vi "Problem 15 - backtracking-optimised.vi"(8 "error in (no error)":errorcluster) -> (0 "error out":errorcluster)   [LabVIEW 2021, in "Project Euler.lvlib"]
uses:
  Project Euler.lvlib
  lattice_path_node.ctl
  lattice_path_direction.ctl
  Utilities/Named Timers/Named Timers.lvlib
panel:
  out "no_of_routes":i32
  out "destination":T1={"position"={"i"=2, "j"=2}, "unexplored children"=[]}
  in  "start":T1={"position"={"i"=0, "j"=0}, "unexplored children"=[enum."to the right", enum."downwards"]}
  out "Loop iteration":i32
  in  "Dev: stop early":bool
  out "no. of columns":i32
  out "no. of rows":i32
  out "map\n2D array of nodes\n(n) x (n) size":T1[][](array[typedef])
  in  "n (number of nodes on a side)":i32=3
  out "Answer":string
  out "Total execution time (ms)":u32
  # "Output\nOutputs of the VI"
  # "Description\n\nBlank VI with error handling case. \n\nSummarize the use of this VI in this space."
  # "Development\ncontrols/indicators useful for development and testing, but which are not outputs of the VI"
  # "Input\nInputs to the VI"
  # "Execution time benchmarking\nFirst implementation:\n\n20x20 grid (21 nodex x 21 nodes):\n125,059 routes found in 506,856 ms -> 4.05 ms to find one route (one average)"
  # "We take n = 8 nodes (grid = 7) as our benchmark.\n\n3,432 routes when n = 8\n\nTime taken (ms)\n\n1. 1100\n2. 1124 \n3. 1116 \n\nimplemented some optimizations\n1. 1038\n2. 1067\n3. 1017\n4. 1017\n5. 1017\n\nimplemented some optimizations:\n- stop if backtracked to start node. This is expected to half execution time.\n1. 521\n2. 527\n3. 517\n4. 533\n5. 519\n\nimplemented some optimizations:\n- restarted LabVIEW after it hanged\n- replaced \"Delete Array Element\" with \"Index Array Subset\"\n1. 71\n2. 78\n3. 82\n4. 77\n5. 66\n\n- replaced \"Index Array Subset\" with \"Delete Array Element\" (back). DAE is faster than ASB in this case.\n1. 51 \n2. 44\n3. 52\n4. 53\n5. 55\n- implemented \"In Place Element Structure\" inside \"find next node.vi\". This subVI executes every iteration of the while loop, so may have a significant effect (10% decrease in exec time). Actual measurements:\n1. 448\n2. 457\n3. 468\n4. 460\n5. 450\n- restarted LabVIEW. Restarting LabVIEW has the single biggest effect on exec time. Why?\n1. 57\n2. 48\n3. 48\n4. 60\n5. 49"
  # "n = 9; 168 ms\nn= 10; 616 ms\nn =11; 2,336; non-optimised time = 8,807. Four-fold optimisation (two-fold in one go, the other factor of two compounded from several optimisations)\n\nn =12; 9119; 705,432 routes\nn =13;\n\nn=14; finished;\n10,400,600 found in 145,041 ms\nAverage: 71.71 routes per ms\n\n----\n\nn=21; stopped early.\n40,014,690 routes found (40 million)\nin\n1,458,759 ms (24.3 minutes)\nAverage: 27.43 routes found per millisecond"
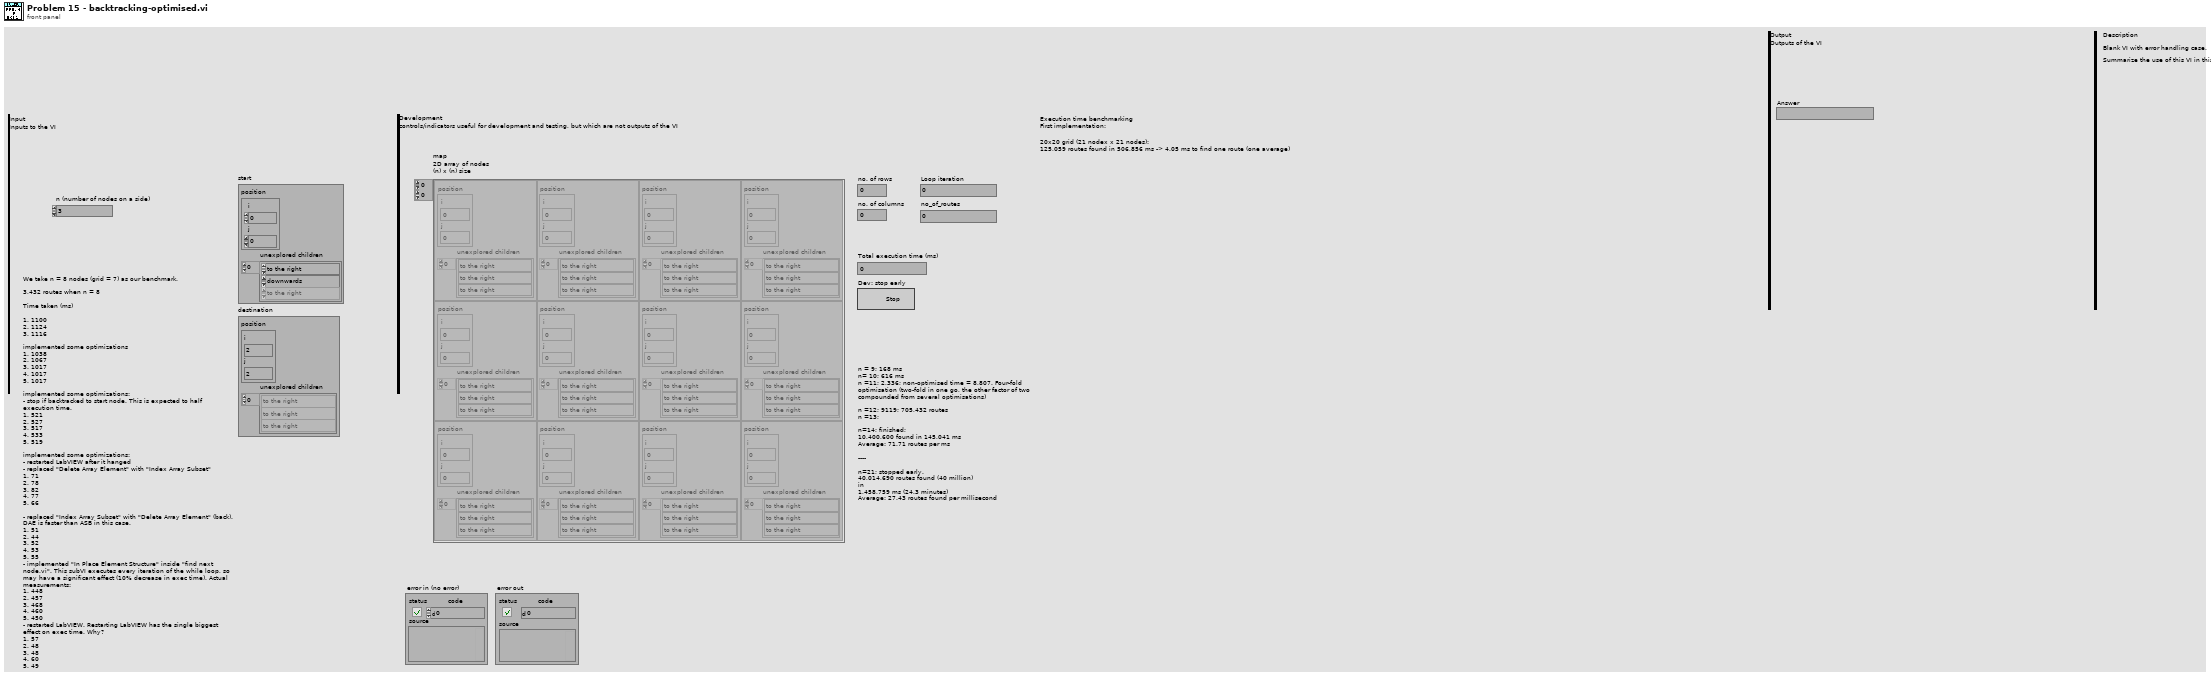
[diagram p1: front panel]
types:
  T1 = typedef "Project Euler.lvlib/lattice_path_node.ctl" = cluster{"position":cluster{"i":i32, "j":i32}, "unexplored children":T2[]}
  T2 = typedef "Project Euler.lvlib/lattice_path_direction.ctl" = enum16{"to the right", "downwards"}
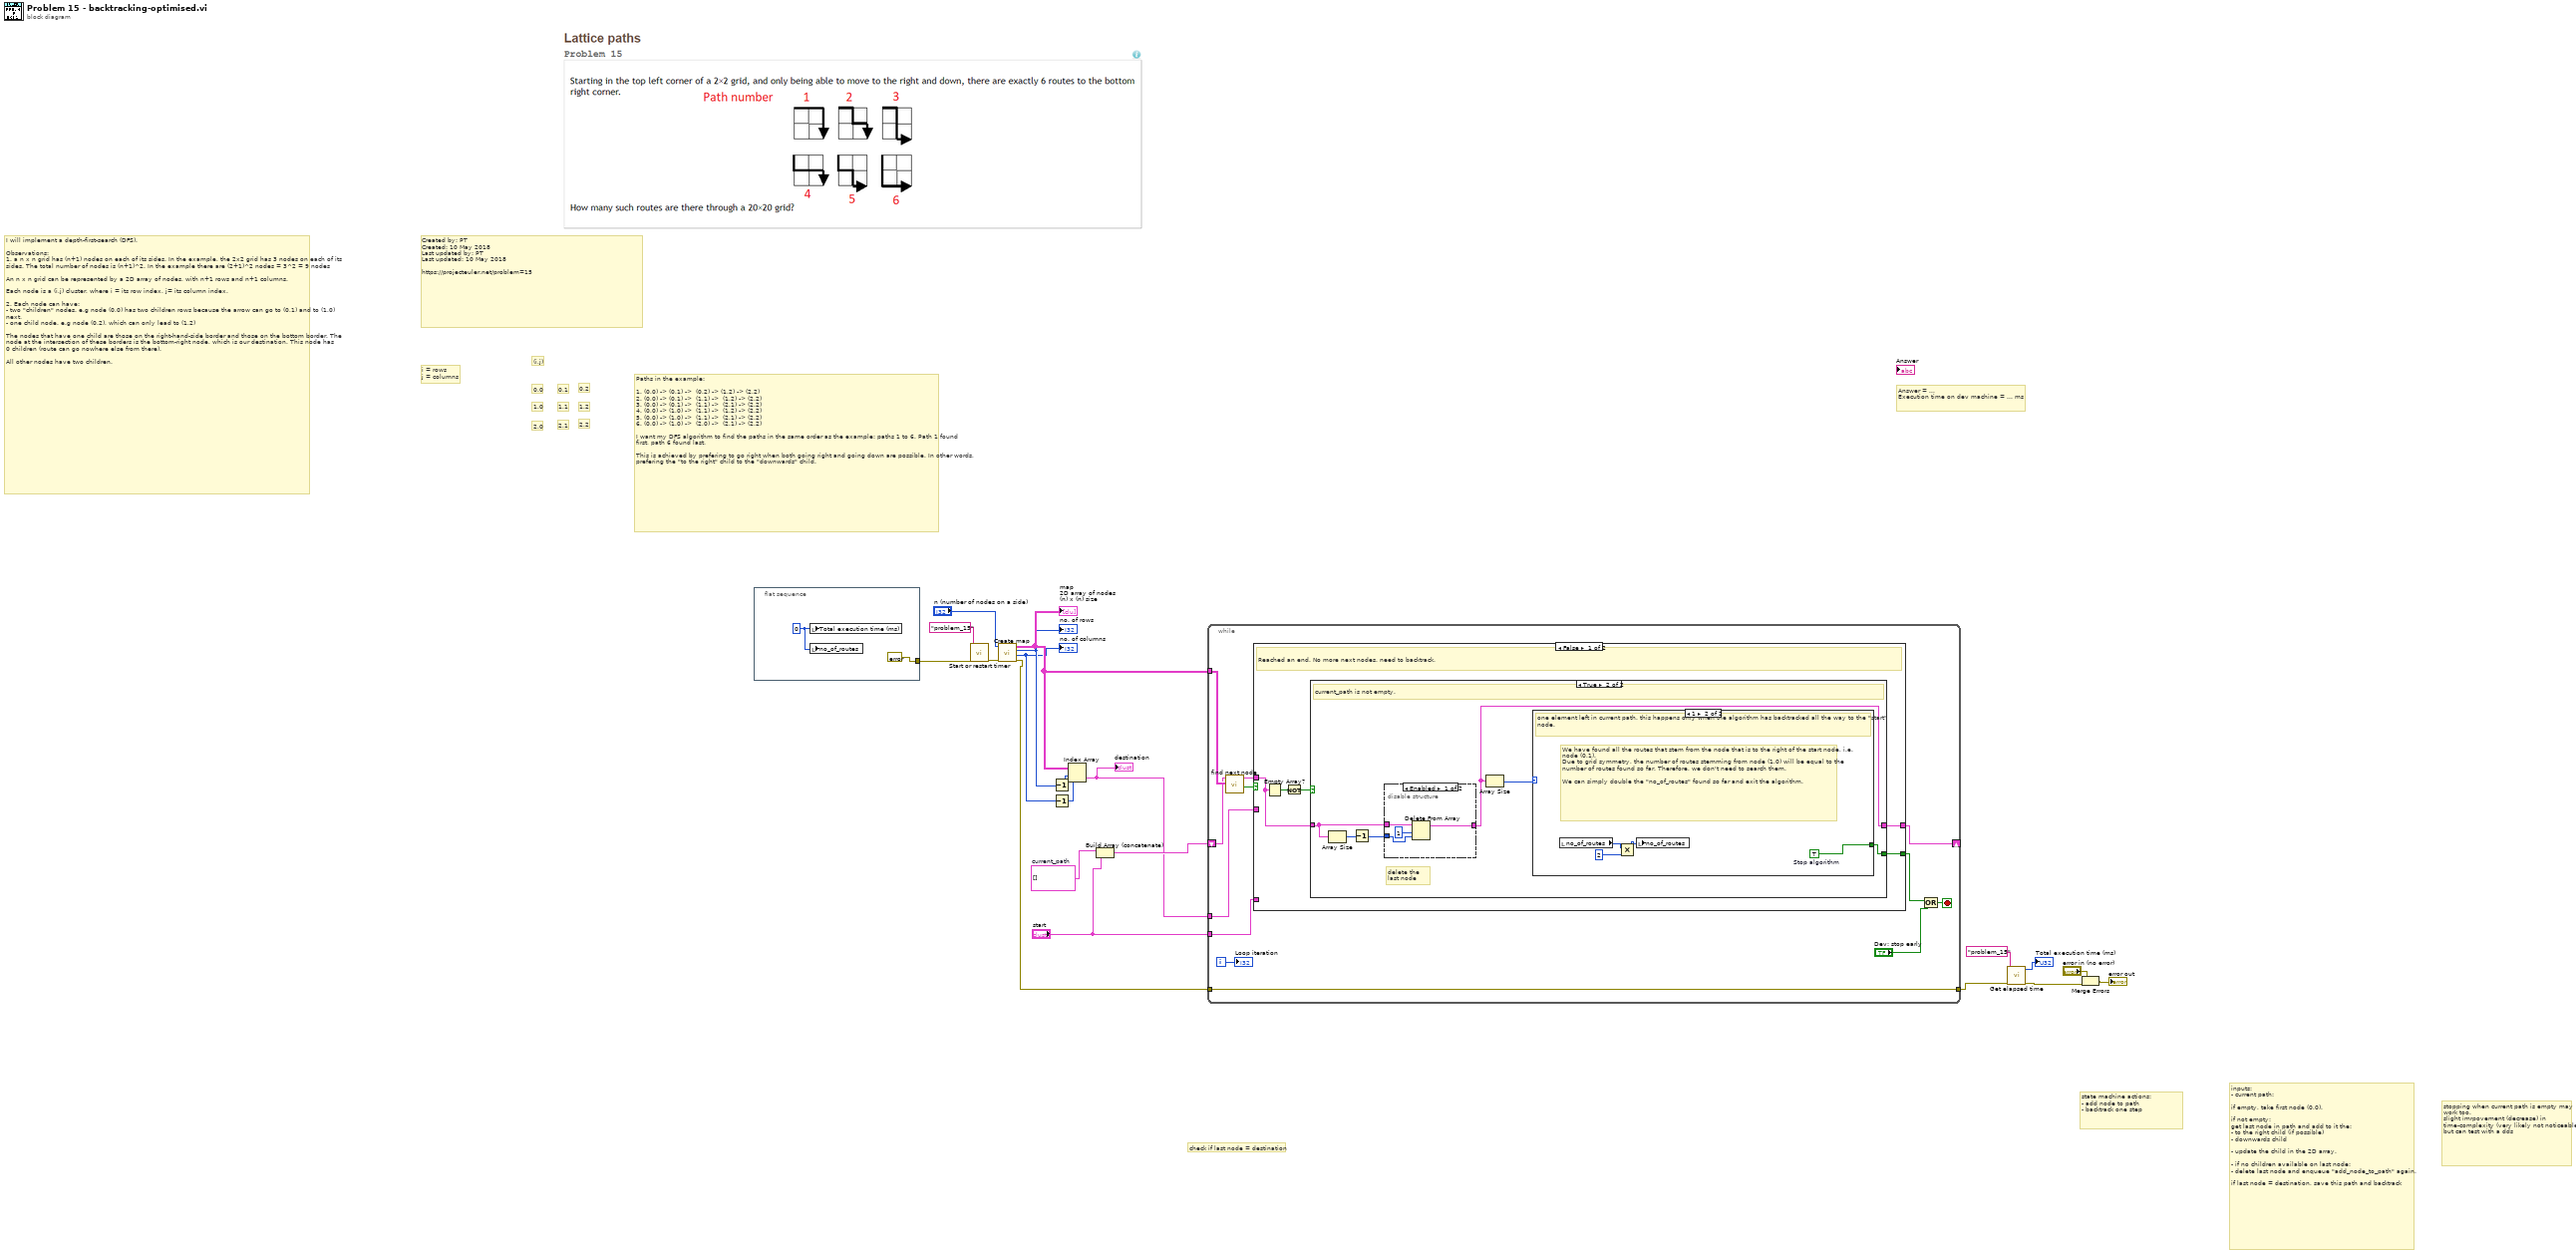
[diagram p0: block diagram]
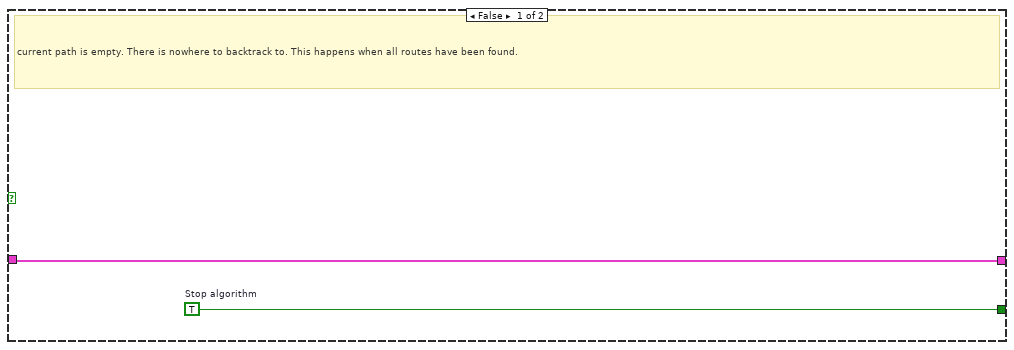
[diagram p2: hidden frame]
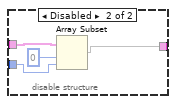
[diagram p3: hidden frame]
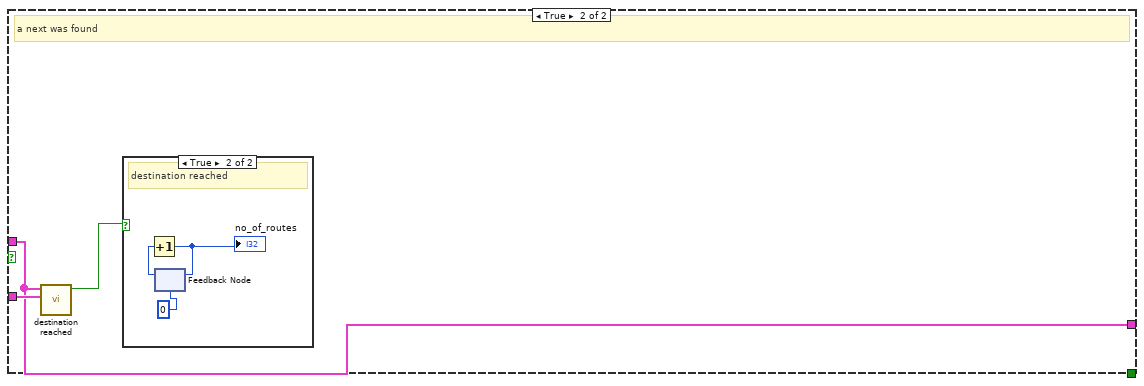
[diagram p5: hidden frame]
diagram:
  w16 = T1[] []  # current_path
  # "stopping when current path is empty may work too.\nslight imrpovement (decrease) in time-complexity (very likely not noticeable), but can test with a dds"
  # "check if last node = destination"
  # "inputs:\n- current path:\n\nif empty, take first node (0,0).\n\nif not empty:\nget last node in path and add to it the:\n- to the right child (if possible)\n- downwards child\n\n- update the child in the 2D array.\n\n- if no children available on last node:\n- delete last node and enqueue \"add_node_to_path\" again.\n\nif last node = destination, save this path and backtrack"
  # "state machine actions:\n- add node to path\n- backtrack one step"
  # "Paths in the example:\n\n1. (0,0) -> (0,1) ->  (0,2) -> (1,2) -> (2,2)\n2. (0,0) -> (0,1) ->  (1,1) ->  (1,2) -> (2,2)\n3. (0,0) -> (0,1) ->  (1,1) ->  (2,1) -> (2,2)\n4. (0,0) -> (1,0) ->  (1,1) ->  (1,2) -> (2,2)\n5. (0,0) -> (1,0) ->  (1,1) ->  (2,1) -> (2,2)\n6. (0,0) -> (1,0) ->  (2,0) ->  (2,1) -> (2,2)\n\nI want my DFS algorithm to find the paths in the same order as the example: paths 1 to 6. Path 1 found first, path 6 found last.\n\nThis is achieved by prefering to go right when both going right and going down are possible. In other words, prefering the \"to the right\" child to the \"downwards\" child."
  # "2,2"
  # "2,1"
  # "1,2"
  # "1,1"
  # "0,2"
  # "0,1"
  # "2,0"
  # "(i,j)"
  # "i = rows\nj = columns"
  # "1,0"
  # "0,0"
  # "I will implement a depth-first-search (DFS).\n\nObservations:\n1. a n x n grid has (n+1) nodes on each of its sides. In the example, the 2x2 grid has 3 nodes on each of its sides. The total number of nodes is (n+1)^2. In the example there are (2+1)^2 nodes = 3^2 = 9 nodes\n\nAn n x n grid can be represented by a 2D array of nodes, with n+1 rows and n+1 columns.\n\nEach node is a (i,j) cluster, where i = its row index, j= its column index.\n\n2. Each node can have:\n- two \"children\" nodes. e.g node (0,0) has two children rows because the arrow can go to (0,1) and to (1,0) next.\n- one child node. e.g node (0,2), which can only lead to (1,2)\n\nThe nodes that have one child are those on the right-hand-side border and those on the bottom border. The node at the intersection of these borders is the bottom-right node, which is our destination. This node has 0 children (route can go nowhere else from there).\n\nAll other nodes have two children."
  # "Answer = ... \nExecution time on dev machine = ... ms"
  # "Created by: PT\nCreated: 10 May 2018\nLast updated by: PT\nLast updated: 10 May 2018\n\nhttps://projecteuler.net/problem=15"
  n1 = flat-sequence {
    tunnel: [w22] -> _
    tunnel: [w22] -> w17
    frame #0 {
      w22 = errorcluster {"status"=FALSE, "code"=0, "source"=""} ("error constant")
      w21 = u32 0 ("Total execution time (ms)")
      n2 = local write "Total execution time (ms)"(w21) -> ()
      n3 = local write "no_of_routes"(w21) -> ()
    }
  }
  n4 = call "Start or restart timer.vi"("error in (no error)"=w17, "Timer name"="problem_15") -> ("error out"=w6:errorcluster)  [unwired: 9 in]
  n5 = call "Create map.vi"("error in (no error)"=w6, "n (number of nodes on a side)"="n (number of nodes on a side)") -> ("error out"=w3:errorcluster, "no. of columns"=w4:i32, "no. of rows"=w5:i32, "map\n2D array of nodes\n(n) x (n) size"=w8:T1[][])  [unwired: 6 in]
  "map\n2D array of nodes\n(n) x (n) size" <- w8
  "no. of rows" <- w5
  "no. of columns" <- w4
  n6 = Decrement(x=w5) -> (x-1=w11:i32)
  n7 = Decrement(x=w4) -> (x-1=w10:i32)
  n8 = Index Array(array=w8, index (row)=w11, index (col)=w10) -> (element=w9:T1)
  "destination" <- w9
  n9 = Build Array (concatenate)(w16, "start") -> (w12:T1[])
  n10 = while {
    shift-right: [w28] -> _
    shift-left: w12 -> [w30]
    tunnel: w8 -> [w31]
    tunnel: w9 -> [w29]
    tunnel: w3 -> [w24]
    tunnel: [w24] -> w2
    tunnel: "start" -> [w23]
    i -> [w32]
    stop <- w33 stop-if-true
    n11 = call "find next node.vi"("map"=w31, "current_path in"=w30) -> ("T = a next node was found"=w26:bool, "current_path out"=w25:T1[])  [unwired: 6 in, 2 out]
    n12 = case shown="False" w26 {
      tunnel: w25 -> [w37 w60]
      tunnel: w29 -> [_ w61]
      tunnel: [w36 _] -> w27
      tunnel: [w35 w60] -> w28
      tunnel: w23 -> [_ _]
      frame False {
        # "Reached an end. No more next nodes. need to backtrack."
        n13 = Empty Array?(array=w37) -> (empty?=w39:bool)
        n14 = Not(x=w39) -> (.not. x?=w38:bool)
        n15 = case shown="True" w38 {
          tunnel: w37 -> [w41 w43]
          tunnel: [w41 w45] -> w35
          tunnel: [w40 w44] -> w36
          frame False {
            w40 = TRUE  # Stop algorithm
            # "current path is empty. There is nowhere to backtrack to. This happens when all routes have been found."
          }
          frame True {
            # "delete the last node"
            # "current_path is not empty."
            n16 = Array Size(array=w43) -> (size(s)=w47:i32)
            n17 = Decrement(x=w47) -> (x-1=w42:i32)
            n18 = disable-structure shown="Enabled" {
              disable-tunnel: [w50 w53] -> w45
              disable-tunnel: w43 -> [w49 w54]
              disable-tunnel: w42 -> [w48 w52]
              frame Enabled {
                n19 = Delete From Array "Delete From Array"(array=w49, length=1, index=w48) -> (array with subset deleted=w50:T1[])  [unwired: 1 out]
              }
              frame Disabled {
                n20 = Array Subset(array=w54, index=0, length=w52) -> (w53:T1[])
              }
            }
            n21 = Array Size(array=w45) -> (size(s)=w46:i32)
            n22 = case shown="1" w46 {
              tunnel: [_ w59] -> w44
              frame Default {
                # "we have not backtracked to the \"start\" node yet"
              }
              frame 1 {
                w59 = TRUE  # Stop algorithm
                # "We have found all the routes that stem from the node that is to the right of the start node, i.e. node (0,1).\nDue to grid symmetry, the number of routes stemming from node (1,0) will be equal to the number of routes found so far. Therefore, we don't need to search them.\n\nWe can simply double the \"no_of_routes\" found so far and exit the algorithm."
                # "one element left in current path. this happens only when the algorithm has backtracked all the way to the \"start\" node."
                n23 = local read "no_of_routes"() -> (w58:i32)
                n24 = Multiply(x=w58, y=2) -> (x*y=w56:i32)
                n25 = local write "no_of_routes"(w56) -> ()
              }
            }
          }
        }
      }
      frame True {
        # "a next was found"
        n26 = call "destination reached.vi"("destination"=w61, "current_path"=w60) -> ("T = destination has been reached"=w62:bool)  [unwired: 8 in, 1 out]
        n27 = case shown="True" w62 {
          frame False {
            # "destination not reached yet"
          }
          frame True {
            # "destination reached"
            n28 = feedback #1(0) -> (w65:i32)
            n29 = Increment(x=w65) -> (x+1=w64:i32)
            "no_of_routes" <- w64
            n30 = feedback-in #1(w64) -> ()
          }
        }
      }
    }
    n31 = Compound Arithmetic op=OR(w27, "Dev: stop early") -> (w33:bool)
    "Loop iteration" <- w32
  }
  n32 = call "Get elapsed time.vi"("error in (no error)"=w2, "Timer name"="problem_15") -> ("error out"=w13:errorcluster, "Elapsed time (ms)"=→"Total execution time (ms)":u32)  [unwired: 6 in, 2 out]
  n33 = Merge Errors("error in (no error)", w13) -> (→"error out":errorcluster)
